vi "CATPLAT GUI.vi"() -> ()   [LabVIEW 2015]
uses:
  controls/PS3 Controls.ctl
  controls/UDP Message Data.ctl
  <vilib>/Utility/error.llb/DialogType.ctl
  <vilib>/Analysis/baseanly.llb/Mean (DBL).vi
  <vilib>/Instr/_visa.llb/VISA Configure Serial Port (Instr).vi
  <vilib>/Instr/_visa.llb/VISA Configure Serial Port (Serial Instr).vi
  <vilib>/Utility/inputDevices.llb/closeJoystick.vi
  <vilib>/regexp/Match Regular Expression.xnode
  <vilib>/Analysis/NI_AALBase.lvlib
panel:
  out "Change PWM":bool
  out "Serial Ports Number":u32
  out "semSocket":T1
  in  "Send ACK":bool
  out "semQueue":T1
  out "UDP Socket":refnum<k16>
  in  "Tab Control":T2(tab)
  out "PWM Indicator":bool caption="PWM"
  out "Speed & Direction":bool
  out "Differential Drive":bool
  out "Righ Caterpillar Speed PWM":i16 caption="Sent Speed Order"
  in  "Right Caterpillar Direction":enum16{"Stop", "Forwards", "Backwards"}(ring) caption="Direction"
  out "Righ Caterpillar Speed":dbl caption="Rcv Speed (m/s)"
  out "Left Caterpillar Speed PWM":i16 caption="Sent Speed Order"
  in  "Left Caterpillar Direction":enum16{"Stop", "Forwards", "Backwards"}(ring) caption="Direction"
  out "Left Caterpillar Speed":dbl caption="Rcv Speed (m/s)"
  out "Sent Exit Command":bool
  in  "Controller Mode":u16(ring) items=["Differential Drive", "Speed & Direction"]
  in  "Exit CATPLAT":bool
  out "CATPLAT Speed (m/s)":dbl(knob) scale=0.0..0.1
  in  "Communication Link":bool
  out "User controller":bool
  out "WiFi Network":bool
  out "UDP Socket":bool
  out "Serial Communication":bool
  in  "stop":bool
  in  "Request Battery":bool
  out "Message received":bool
  out "Error Out":errorcluster
  in  "restart":bool
  out "Battery level":u8(slide) scale=0.0..100.0
  out "rvcMsgs":refnum<queue>
  in  "No. Pulses":i32=8
  in  "Diameter (mm)":i32=10
  in  "PWM":bool
  in  "Threshold":i32=25000
  in  "Message Type":T3(ring)
  out "Change Controller Mode":bool
  in  "Update":bool
  in  "Password":string="caterpillarPlatform"
  in  "SSID":string="caterpillarWiFi"
  in  "Computer  IP":string
  in  "Computer Port":u16=3000
  in  "Platform IP":string
  in  "Platform Port":u16
  out "Left Joystick X Axis":i32
  out "Left Joystick Y Axis":i32
  out "Right Joystick X Axis":i32
  out "Right Joystick Y Axis":i32
  out "PS3 Controls":T4 {"Left Analogue Stick X" scale=-32768.0..32768.0; "Left Analogue Stick Y" scale=32768.0..-32768.0; "Right Analogue Stick X" scale=-32768.0..32768.0; "Right Analogue Stick Y" scale=32768.0..-32768.0; "X Rotation" scale=-32768.0..32768.0; "Y Rotation" scale=-32768.0..32768.0; "L2 Pressure" scale=0.0..32768.0; "Numeric" format="%d°"}
  in  "All Logs":bool
  in  "Clear Log":bool
  in  "Autoscroll":bool=TRUE
  in  "Log":string
  in  "Clear Log Serial":bool
  in  "Autoscroll Serial":bool=TRUE caption="Autoscroll"
  in  "Baud Rate":u32=115200
  in  "Serial Port List":refnum<visa-resource-name>
  in  "Serial log":string
  out "Controller":refnum<k1>
  # "Controls"
  # "Right Caterpillar"
  # "Left Caterpillar"
  # "Errors"
  # "Information"
  # "Controller Settings"
  # "Encoder Settings"
  # "WiFi Network Settings"
  # "UDP Settings"
  # "CATPLAT GUI Log"
  # "CATPLAT Log"
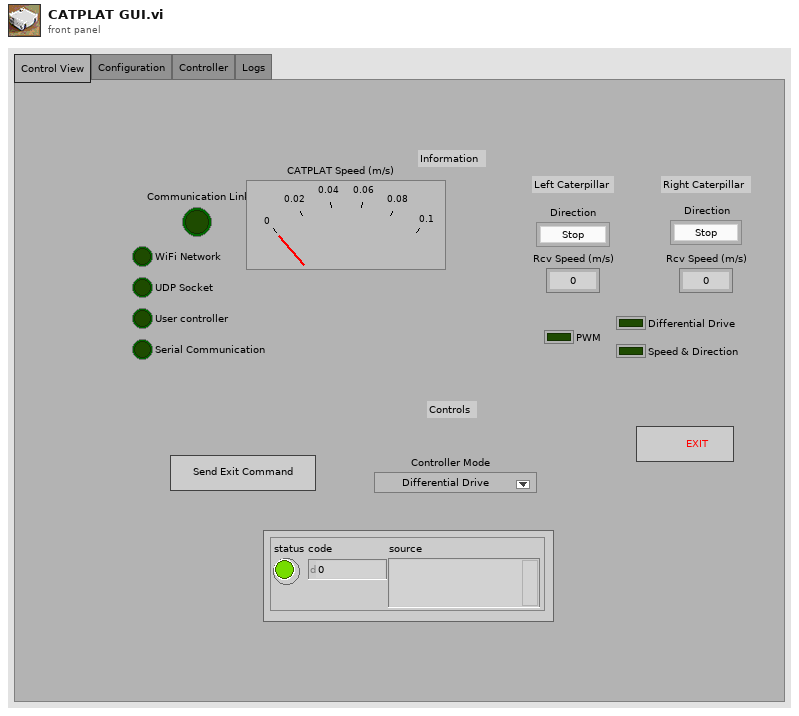
[diagram p1: front panel]
types:
  T1 = typedef "Semaphore RefNum" = refnum<k1>
  T2 = enum32{"Control View", "Configuration", "Controller", "Logs"}
  T3 = enum16{"Acknowledge", "Speed", "Brake", "Watchdog", "Update", "Exit", "Init", "Log", "Unknown"}
  T4 = typedef "PS3 Controls.ctl" = cluster{"Left Analogue Stick X":i32, "Left Analogue Stick Y":i32, "Right Analogue Stick X":i32, "Right Analogue Stick Y":i32, "Y Rotation":i32, "X Rotation":i32, "L2 Pressure":i32, "R2 Pressure":i32, "Triangle":bool, "Circle":bool, "X":bool, "Square":bool, "L1":bool, "R1":bool, "L2":bool, "R2":bool, "L3":bool, "R3":bool, "Select":bool, "Start":bool, "PS Button":bool, "Numeric":i32}
  T5 = enum8{"Enabled", "Disabled", "Disabled and Grayed Out"}
  T6 = typedef "UDP Message Data.ctl" = cluster{"Command":enum16{"Acknowledge", "Speed", "Brake", "Watchdog", "Update", "Exit", "Init", "Log", "Unknown"}, "Msg Length":u8, "Content Bytes":u8[], "Content String":string, "CRC8":u8, "Valid?":bool}
  T7 = typedef "DialogType.ctl" = u16
  T8 = enum32{"invalid app kind", "Development System", "Run Time System", "Student Edition", "Embedded LabVIEW", "Evaluation", "Custom"}
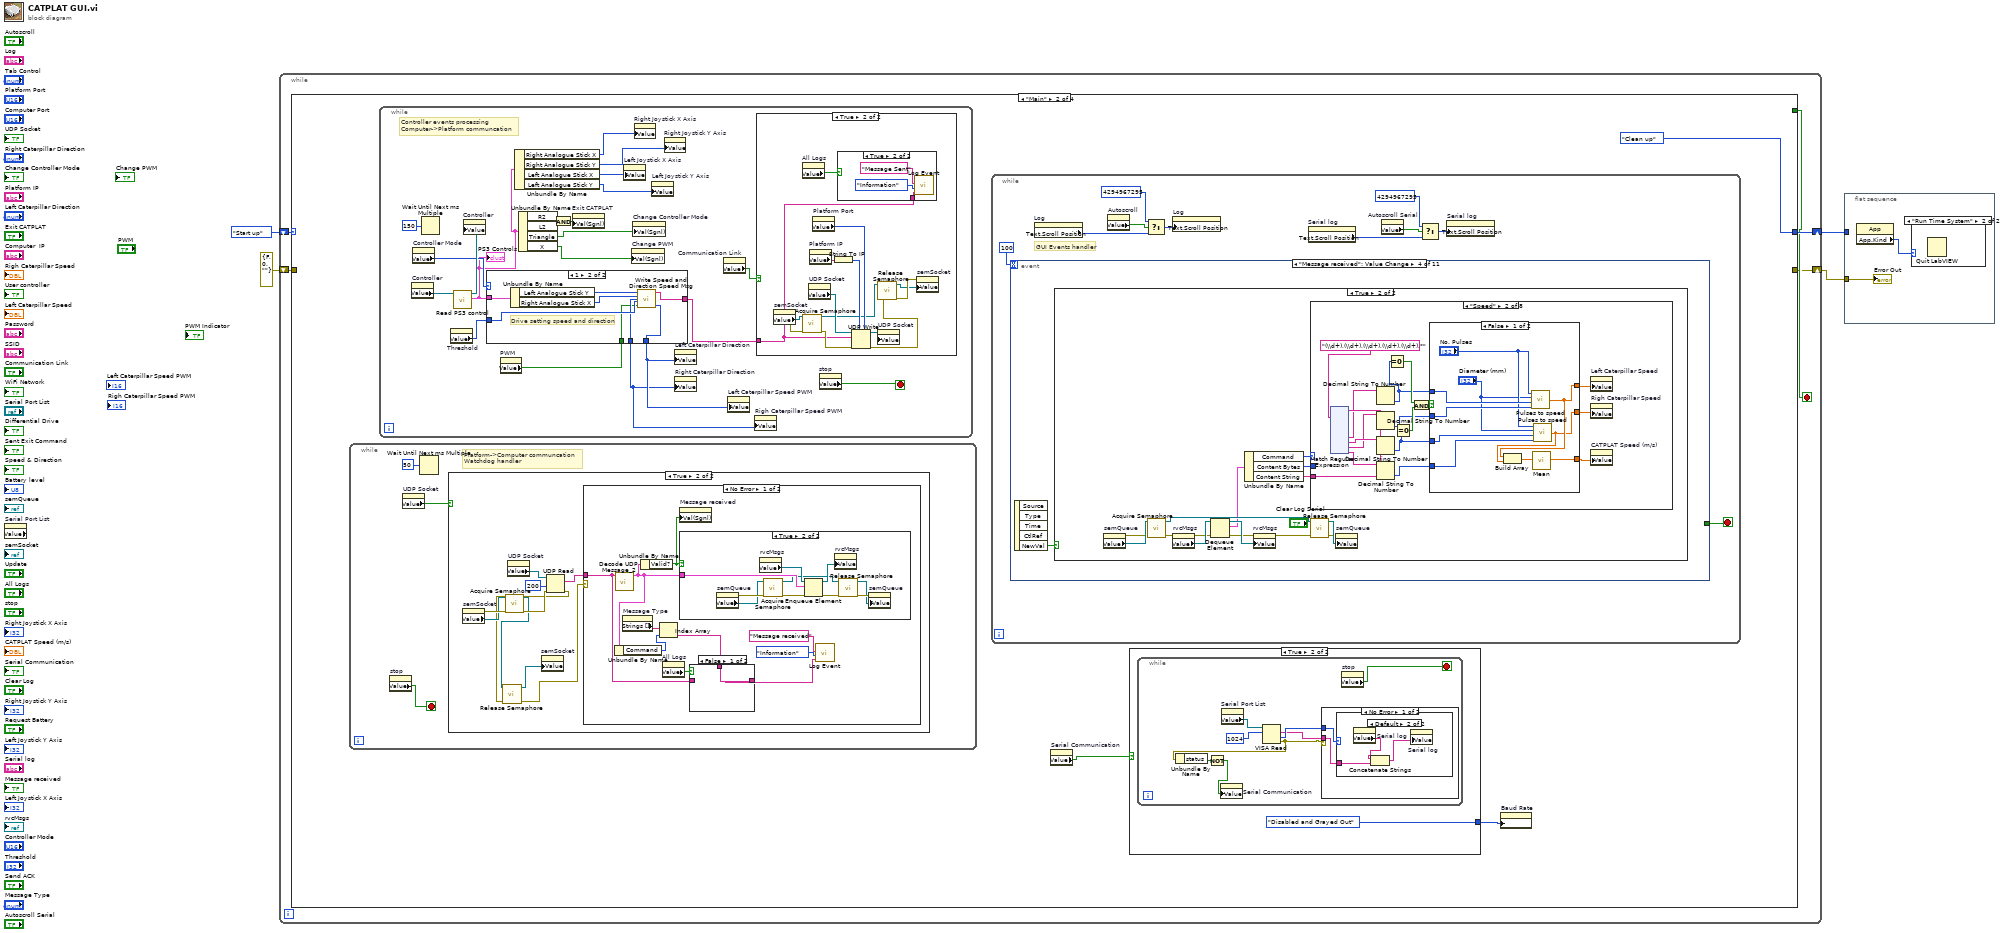
[diagram p0: block diagram]
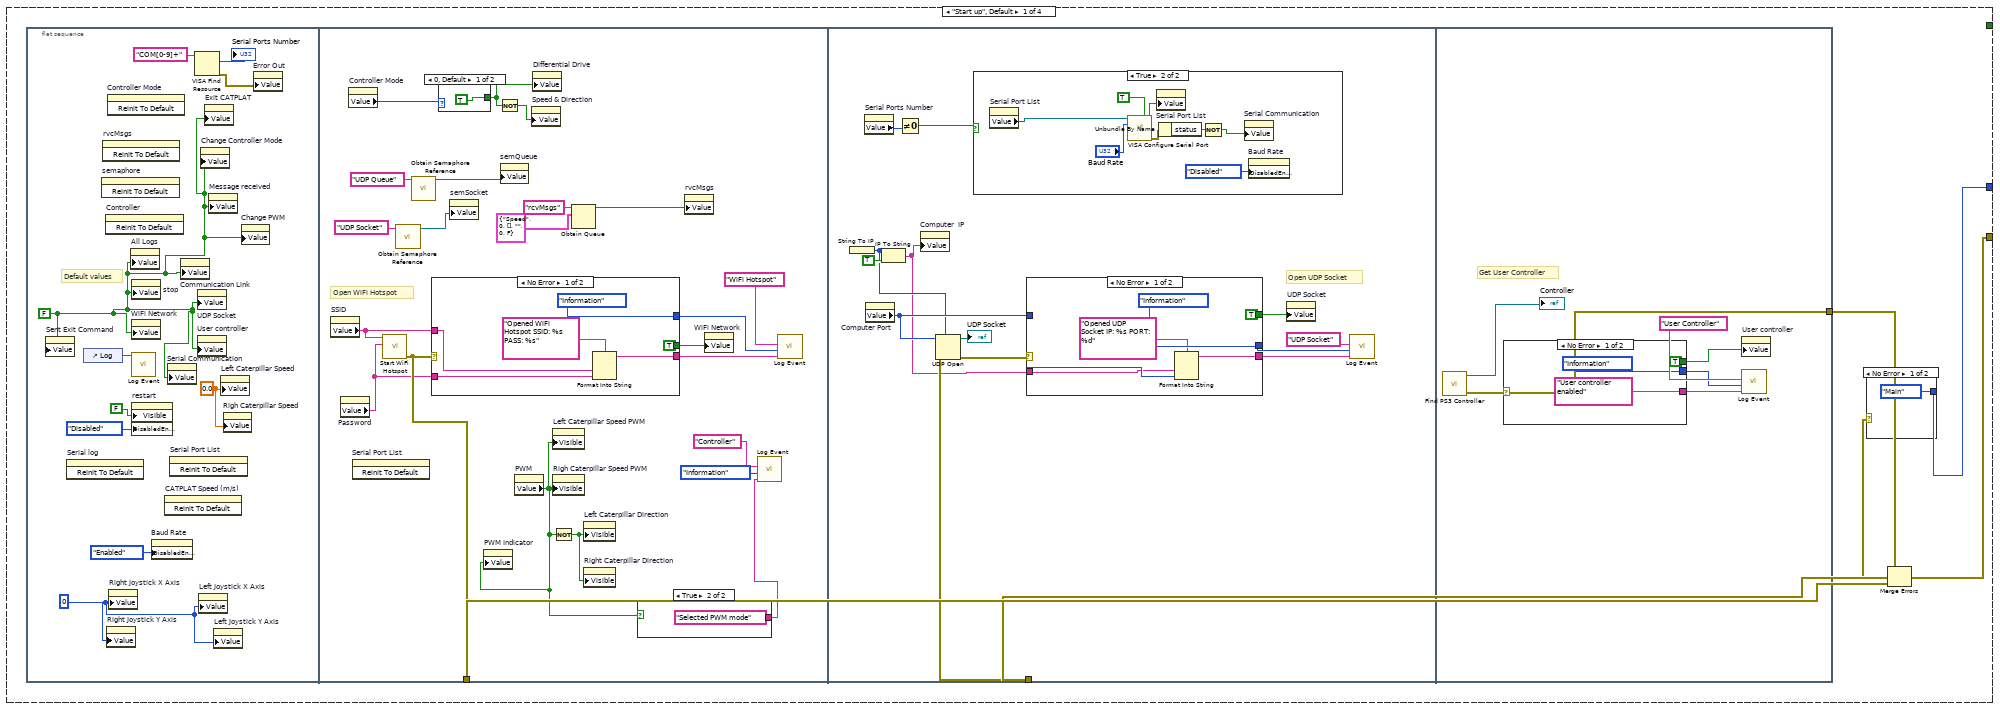
[diagram p3: hidden frame]
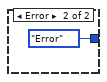
[diagram p4: hidden frame]
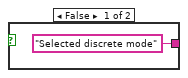
[diagram p5: hidden frame]
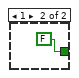
[diagram p6: hidden frame]
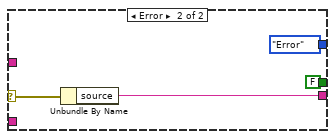
[diagram p7: hidden frame]
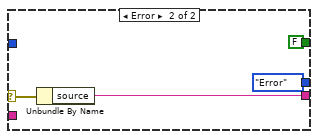
[diagram p9: hidden frame]
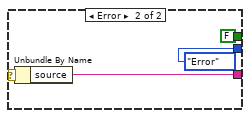
[diagram p10: hidden frame]
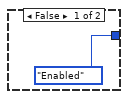
[diagram p11: hidden frame]
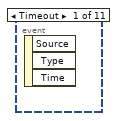
[diagram p14: hidden frame]
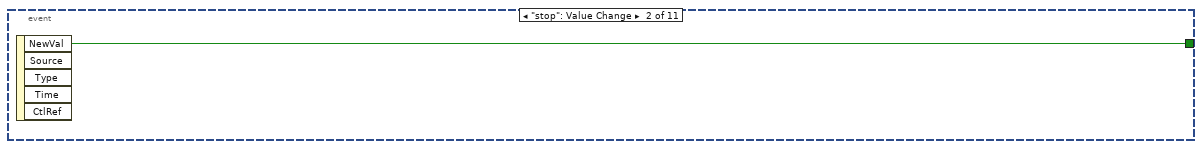
[diagram p15: hidden frame]
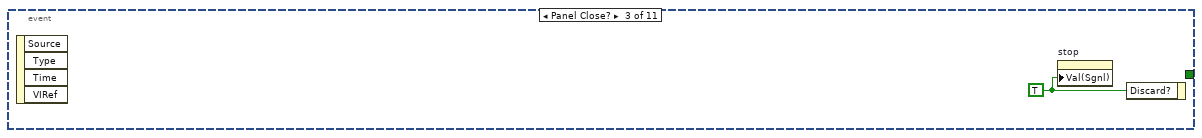
[diagram p16: hidden frame]
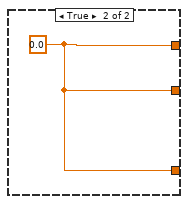
[diagram p19: hidden frame]
diagram:
  n1 = property on="Serial Port List" class="VISAName" props=["Value"]() -> ()  [unwired: 2 in, 3 out]
  n2 = while {
    shift-right: [w8] -> w3
    shift-left: enum16{"Start up", "Error", "Main", "Clean up"}."Start up" -> [w9]
    shift-right: [w6] -> w2
    shift-left: errorcluster {"status"=FALSE, "code"=0, "source"=""} ("error IO") -> [w5]
    stop <- w7 stop-if-true
    n3 = case shown="\"Main\"" w9 {
      selector: w9 -> [_ _ w634 _]
      tunnel: [w14 enum16{"Start up", "Error", "Main", "Clean up"}."Clean up" w634 w641] -> w8
      tunnel: [_ _ TRUE _] -> w7
      tunnel: [w10 _ w628 errorcluster {"status"=FALSE, "code"=0, "source"=""} ("error IO")] -> w6
      tunnel: w5 -> [_ _ w627 w640]
      frame "Start up", Default {
        n4 = flat-sequence {
          tunnel: [w48] -> w12
          tunnel: [w73] -> w11
          tunnel: [w93] -> w13
          frame #0 {
            w18 = i64 0 ("Right Joystick X Axis")
            w23 = 0.0 ("Left wheel speed")
            w17 = FALSE ("stop")
            # "Default values"
            n5 = property on="Sent Exit Command" class="Bool (strict)"("Value"=w17) -> ()  [unwired: 2 in, 2 out]
            n6 = invoke on="Serial log" class="Str" method="Reinit To Default"() -> ()  [unwired: 3 in, 3 out]
            n7 = control-ref of="Log"() -> (w24:refnum<vi>)
            n8 = invoke on="semaphore" class="TypRef (strict)" method="Reinit To Default"() -> ()  [unwired: 3 in, 3 out]
            n9 = invoke on="rvcMsgs" class="TypRef (strict)" method="Reinit To Default"() -> ()  [unwired: 3 in, 3 out]
            n10 = invoke on="Controller" class="TypRef (strict)" method="Reinit To Default"() -> ()  [unwired: 3 in, 3 out]
            n11 = property on="Right Joystick Y Axis" class="DigNum (strict)"("Value"=w18) -> ()  [unwired: 2 in, 2 out]
            n12 = invoke on="Controller Mode" class="Ring (strict)" method="Reinit To Default"() -> ()  [unwired: 3 in, 3 out]
            n13 = property on="Right Joystick X Axis" class="DigNum (strict)"("Value"=w18) -> ()  [unwired: 2 in, 2 out]
            n14 = property on="All Logs" class="Bool (strict)"("Value"=w17) -> ()  [unwired: 2 in, 2 out]
            n15 = property on="stop" class="Bool (strict)"("Value"=w17) -> ()  [unwired: 2 in, 2 out]
            n16 = property on="WiFi Network" class="Bool (strict)"("Value"=w17) -> ()  [unwired: 2 in, 2 out]
            n17 = call "Log Event.vi"("Log Refnum"=w24) -> ()  [unwired: 11 in]
            n18 = property on="restart" class="Bool (strict)"("Visible"=FALSE, "DisabledEnum"=T5."Disabled" ("Disabled")) -> ()  [unwired: 2 in, 2 out]
            n19 = property on="Baud Rate" class="DigNum (strict)"("DisabledEnum"=T5."Enabled" ("Disabled")) -> ()  [unwired: 2 in, 2 out]
            n20 = invoke on="CATPLAT Speed (m/s)" class="Knob (strict)" method="Reinit To Default"() -> ()  [unwired: 3 in, 3 out]
            n21 = property on="Serial Communication" class="Bool (strict)"("Value"=w17) -> ()  [unwired: 2 in, 2 out]
            n22 = invoke on="Serial Port List" class="VISAName" method="Reinit To Default"() -> ()  [unwired: 3 in, 3 out]
            n23 = property on="Communication Link" class="Bool (strict)"("Value"=w17) -> ()  [unwired: 2 in, 2 out]
            n24 = VISA Find Resource(11:"COM[0-9]+" ("expression (\"?*\")")) -> (0:w20:errorcluster, 2:→"Serial Ports Number":u32)  [unwired: 2 in, 1 out]
            n25 = property on="UDP Socket" class="Bool (strict)"("Value"=w17) -> ()  [unwired: 2 in, 2 out]
            n26 = property on="User controller" class="Bool (strict)"("Value"=w17) -> ()  [unwired: 2 in, 2 out]
            n27 = property on="Left Joystick X Axis" class="DigNum (strict)"("Value"=w18) -> ()  [unwired: 2 in, 2 out]
            n28 = property on="Change Controller Mode" class="Bool (strict)"("Value"=w17) -> ()  [unwired: 2 in, 2 out]
            n29 = property on="Exit CATPLAT" class="Bool (strict)"("Value"=w17) -> ()  [unwired: 2 in, 2 out]
            n30 = property on="Message received" class="Bool (strict)"("Value"=w17) -> ()  [unwired: 2 in, 2 out]
            n31 = property on="Left Joystick Y Axis" class="DigNum (strict)"("Value"=w18) -> ()  [unwired: 2 in, 2 out]
            n32 = property on="Left Caterpillar Speed" class="DigNum (strict)"("Value"=w23) -> ()  [unwired: 2 in, 2 out]
            n33 = property on="Righ Caterpillar Speed" class="DigNum (strict)"("Value"=w23) -> ()  [unwired: 2 in, 2 out]
            n34 = property on="Change PWM" class="Bool (strict)"("Value"=w17) -> ()  [unwired: 2 in, 2 out]
            n35 = property on="Error Out" class="Clust (strict)"("Value"=w20) -> ()  [unwired: 2 in, 2 out]
          }
          frame #1 {
            # "Open WiFi Hotspot"
            n36 = property on="SSID" class="Str"() -> ("Value"=w46:string)  [unwired: 2 in, 2 out]
            n37 = property on="Password" class="Str"() -> ("Value"=w45:string)  [unwired: 2 in, 2 out]
            n38 = property on="Controller Mode" class="Ring (strict)"() -> ("Value"=w34:u16)  [unwired: 2 in, 2 out]
            n39 = invoke on="Serial Port List" class="VISAName" method="Reinit To Default"() -> ()  [unwired: 3 in, 3 out]
            n40 = call "Start WiFi Hotspot.vi"("Password"=w45, "SSID"=w46) -> ("error out"=w48:errorcluster)  [unwired: 9 in]
            n41 = call <vilib>:"Obtain Semaphore Reference.vi"("name (unnamed)"="UDP Socket") -> ("semaphore"=w35:T1)  [unwired: 4 in, 2 out]
            n42 = call <vilib>:"Obtain Semaphore Reference.vi"("name (unnamed)"="UDP Queue") -> ("semaphore"=w36:T1)  [unwired: 4 in, 2 out]
            n43 = case shown="No Error" w48 {
              selector: w48 -> [_ w61]
              tunnel: [enum16{"Information", "Warning", "Error"}."Information" ("Enum") enum16{"Information", "Warning", "Error"}."Error" ("Enum")] -> w47
              tunnel: w46 -> [w56 _]
              tunnel: w45 -> [w55 _]
              tunnel: [w54 w60] -> w44
              tunnel: [TRUE ("WiFi Network") FALSE ("WiFi Network")] -> w42
              frame No Error {
                n44 = Format Into String(format string="Opened WiFi Hotspot SSID: %s PASS: %s" ("Event"), w56, w55) -> (resulting string=w54:string)  [unwired: 2 in, 1 out]
              }
              frame Error {
                n45 = Unbundle By Name(w61) -> ("source"=w60:string)
              }
            }
            n46 = case shown="0, Default" w34 {
              tunnel: [TRUE FALSE] -> w33
              frame 0, Default {
              }
              frame 1 {
              }
            }
            n47 = property on="semSocket" class="TypRef (strict)"("Value"=w35) -> ()  [unwired: 2 in, 2 out]
            n48 = Not(x=w33) -> (.not. x?=w32:bool)
            n49 = property on="semQueue" class="TypRef (strict)"("Value"=w36) -> ()  [unwired: 2 in, 2 out]
            n50 = property on="PWM" class="Bool (strict)"() -> ("Value"=w27:bool)  [unwired: 2 in, 2 out]
            n51 = property on="PWM Indicator" class="Bool (strict)"("Value"=w27) -> ()  [unwired: 2 in, 2 out]
            n52 = property on="Speed & Direction" class="Bool (strict)"("Value"=w32) -> ()  [unwired: 2 in, 2 out]
            n53 = property on="Differential Drive" class="Bool (strict)"("Value"=w33) -> ()  [unwired: 2 in, 2 out]
            n54 = Not(x=w27) -> (.not. x?=w31:bool)
            n55 = property on="Left Caterpillar Speed PWM" class="DigNum (strict)"("Visible"=w27) -> ()  [unwired: 2 in, 2 out]
            n56 = property on="Righ Caterpillar Speed PWM" class="DigNum (strict)"("Visible"=w27) -> ()  [unwired: 2 in, 2 out]
            n57 = Obtain Queue(name (unnamed)="rcvMsgs", element data type=T6 {"Command"=enum."Speed", "Msg Length"=0, "Content Bytes"=[], "Content String"="", "CRC8"=0, "Valid?"=FALSE} ("Data")) -> (queue out=w40:refnum<queue>)  [unwired: 3 in, 2 out]
            n58 = property on="Left Caterpillar Direction" class="Enum (strict)"("Visible"=w31) -> ()  [unwired: 2 in, 2 out]
            n59 = property on="Right Caterpillar Direction" class="Enum (strict)"("Visible"=w31) -> ()  [unwired: 2 in, 2 out]
            n60 = case shown="True" w27 {
              tunnel: ["Selected discrete mode" ("Event") "Selected PWM mode" ("Event")] -> w28
              frame False {
              }
              frame True {
              }
            }
            n61 = property on="rvcMsgs" class="TypRef (strict)"("Value"=w40) -> ()  [unwired: 2 in, 2 out]
            n62 = property on="WiFi Network" class="Bool (strict)"("Value"=w42) -> ()  [unwired: 2 in, 2 out]
            n63 = call "Log Event.vi"("Event"=w28, "Enum"=enum16{"Information", "Warning", "Error"}."Information", "Process"="Controller") -> ()  [unwired: 9 in]
            n64 = call "Log Event.vi"("Event"=w44, "Enum"=w47, "Process"="WiFi Hotspot") -> ()  [unwired: 9 in]
          }
          frame #2 {
            # "Open UDP Socket"
            n65 = String To IP() -> (0:w66:u32)  [unwired: 1 in]
            n66 = property on="Serial Ports Number" class="DigNum (strict)"() -> ("Value"=w64:u32)  [unwired: 2 in, 2 out]
            n67 = property on="Computer Port" class="DigNum (strict)"() -> ("Value"=w72:u16)  [unwired: 2 in, 2 out]
            n68 = IP To String(1:TRUE ("dot notation? (F)"), 2:w66) -> (0:w65:string)
            n69 = Not Equal To 0?(x=w64) -> (x != 0?=w63:bool)
            n70 = property on="Computer  IP" class="Str"("Value"=w65) -> ()  [unwired: 2 in, 2 out]
            n71 = UDP Open(7:w66, 11:w72) -> (port=→"UDP Socket":refnum<k16>, 0:w73:errorcluster)  [unwired: 3 in, 1 out]
            n72 = case shown="True" w63 {
              frame False {
              }
              frame True {
                n73 = property on="Serial Port List" class="VISAName"() -> ("Value"=w79:refnum<visa-resource-name>)  [unwired: 2 in, 2 out]
                n74 = call-poly "VISA Configure Serial Port"("VISA resource name"=w79, "Enable Termination\nChar (T)"=TRUE ("Enable Termination\nChar (T)"), "baud rate (9600)"="Baud Rate") -> ("VISA resource name out"=w80:refnum<visa-resource-name>, "error out"=w77:errorcluster)  [unwired: 11 in]
                n75 = property on="Serial Port List" class="VISAName"("Value"=w80) -> ()  [unwired: 2 in, 2 out]
                n76 = Unbundle By Name(w77) -> ("status"=w76:bool)
                n77 = Not(x=w76) -> (.not. x?=w75:bool)
                n78 = property on="Serial Communication" class="Bool (strict)"("Value"=w75) -> ()  [unwired: 2 in, 2 out]
                n79 = property on="Baud Rate" class="DigNum (strict)"("DisabledEnum"=T5."Disabled" ("Disabled")) -> ()  [unwired: 2 in, 2 out]
              }
            }
            n80 = case shown="No Error" w73 {
              selector: w73 -> [_ w91]
              tunnel: [enum16{"Information", "Warning", "Error"}."Information" ("Enum") enum16{"Information", "Warning", "Error"}."Error" ("Enum")] -> w70
              tunnel: w72 -> [w85 _]
              tunnel: w65 -> [w84 _]
              tunnel: [w86 w90] -> w71
              tunnel: [TRUE ("UDP Communication") FALSE ("UDP Communication")] -> w68
              frame No Error {
                n81 = Format Into String(format string="Opened UDP Socket IP: %s PORT: %d" ("Event"), w84, w85) -> (resulting string=w86:string)  [unwired: 2 in, 1 out]
              }
              frame Error {
                n82 = Unbundle By Name(w91) -> ("source"=w90:string)
              }
            }
            n83 = property on="UDP Socket" class="Bool (strict)"("Value"=w68) -> ()  [unwired: 2 in, 2 out]
            n84 = call "Log Event.vi"("Event"=w71, "Enum"=w70, "Process"="UDP Socket") -> ()  [unwired: 9 in]
          }
          frame #3 {
            # "Get User Controller"
            n85 = call "Find PS3 Controller.vi"() -> ("error out"=w93:errorcluster, "Controller Reference Out"=→"Controller":refnum<k1>)  [unwired: 10 in]
            n86 = case shown="No Error" w93 {
              selector: w93 -> [_ w104]
              tunnel: [enum16{"Information", "Warning", "Error"}."Information" ("Enum") enum16{"Information", "Warning", "Error"}."Error" ("Enum")] -> w95
              tunnel: ["User controller enabled" ("Event") w103] -> w97
              tunnel: [TRUE ("UDP Communication") FALSE ("UDP Communication")] -> w98
              frame No Error {
              }
              frame Error {
                n87 = Unbundle By Name(w104) -> ("source"=w103:string)
              }
            }
            n88 = property on="User controller" class="Bool (strict)"("Value"=w98) -> ()  [unwired: 2 in, 2 out]
            n89 = call "Log Event.vi"("Event"=w97, "Enum"=w95, "Process"="User Controller") -> ()  [unwired: 9 in]
          }
        }
        n90 = Merge Errors(w13, w11, w12) -> (w10:errorcluster)
        n91 = case shown="No Error" w10 {
          tunnel: [enum16{"Start up", "Error", "Main", "Clean up"}."Main" enum16{"Start up", "Error", "Main", "Clean up"}."Error"] -> w14
          frame No Error {
          }
          frame Error {
          }
        }
      }
      frame "Main" {
        n92 = while {
          stop <- w583 stop-if-true
          # "Platform->Computer communcation\nWatchdog handler"
          n93 = property on="stop" class="Bool (strict)"() -> ("Value"=w583:bool)  [unwired: 2 in, 2 out]
          n94 = property on="UDP Socket" class="Bool (strict)"() -> ("Value"=w585:bool)  [unwired: 2 in, 2 out]
          n95 = Wait Until Next ms Multiple(millisecond multiple=u32 50) -> ()  [unwired: 1 out]
          n96 = case shown="True" w585 {
            frame False {
            }
            frame True {
              n97 = property on="semSocket" class="TypRef (strict)"() -> (error out=w592:errorcluster, "Value"=w591:T1)  [unwired: 2 in, 1 out]
              n98 = call <vilib>:"Acquire Semaphore.vi"("error in (no error)"=w592, "semaphore"=w591) -> ("error out"=w590:errorcluster, "semaphore out"=w588:T1)  [unwired: 3 in, 1 out]
              n99 = property on="UDP Socket" class="Ref (strict)"() -> ("Value"=w595:refnum<k16>)  [unwired: 2 in, 2 out]
              n100 = UDP Read(connection ID=w595, timeout ms (25000)=200, 8:w590) -> (data out=w593:string, error out=w587:errorcluster)  [unwired: 1 in, 3 out]
              n101 = call <vilib>:"Release Semaphore.vi"("error in (no error)"=w587, "semaphore"=w588) -> ("error out"=w586:errorcluster, "semaphore out"=w589:T1)  [unwired: 4 in]
              n102 = property on="semSocket" class="TypRef (strict)"("Value"=w589) -> ()  [unwired: 2 in, 2 out]
              n103 = case shown="No Error" w586 {
                tunnel: w593 -> [w601 _]
                frame No Error {
                  n104 = call "Decode UDP Message_2.vi"("Input string"=w601) -> ("Data"=w597:T6)  [unwired: 10 in]
                  n105 = Unbundle By Name(w597) -> ("Command"=w598:T3)
                  n106 = property on="Message Type" class="Enum (strict)"() -> ("Strings []"=w599:string[])  [unwired: 2 in, 2 out]
                  n107 = Unbundle By Name(w597) -> ("Valid?"=w603:bool)
                  n108 = Index Array(array=w599, index=w598) -> (element=w596:string)
                  n109 = property on="All Logs" class="Bool (strict)"() -> ("Value"=w602:bool)  [unwired: 2 in, 2 out]
                  n110 = property on="Message received" class="Bool (strict)"("Val(Sgnl)"=w603) -> ()  [unwired: 2 in, 2 out]
                  n111 = case shown="True" w603 {
                    tunnel: w597 -> [_ w617]
                    frame False {
                    }
                    frame True {
                      n112 = property on="semQueue" class="TypRef (strict)"() -> (error out=w616:errorcluster, "Value"=w613:T1)  [unwired: 2 in, 1 out]
                      n113 = property on="rvcMsgs" class="TypRef (strict)"() -> ("Value"=w619:refnum<queue>)  [unwired: 2 in, 2 out]
                      n114 = call <vilib>:"Acquire Semaphore.vi"("error in (no error)"=w616, "semaphore"=w613) -> ("error out"=w611:errorcluster, "semaphore out"=w612:T1)  [unwired: 3 in, 1 out]
                      n115 = Enqueue Element(queue=w619, element=w617, error in (no error)=w611) -> (queue out=w618:refnum<queue>, error out=w610:errorcluster)  [unwired: 1 in, 1 out]
                      n116 = property on="rvcMsgs" class="TypRef (strict)"("Value"=w618) -> ()  [unwired: 2 in, 2 out]
                      n117 = call <vilib>:"Release Semaphore.vi"("error in (no error)"=w610, "semaphore"=w612) -> ("error out"=w615:errorcluster, "semaphore out"=w614:T1)  [unwired: 4 in]
                      n118 = property on="semQueue" class="TypRef (strict)"(error in=w615, "Value"=w614) -> ()  [unwired: 1 in, 2 out]
                    }
                  }
                  n119 = case shown="False" w602 {
                    tunnel: w601 -> [_ w609]
                    tunnel: [w606 w609] -> w600
                    tunnel: w596 -> [w606 w607]
                    frame False {
                    }
                    frame True {
                      n120 = Concatenate Strings(w607, ": " ("string"), w609) -> ()  [unwired: 1 out]
                    }
                  }
                  n121 = call "Log Event.vi"("Event"=w600, "Enum"=enum16{"Information", "Warning", "Error"}."Information", "Process"="Message received") -> ()  [unwired: 9 in]
                }
                frame Error {
                }
              }
            }
          }
        }
        n122 = while {
          stop <- w529 stop-if-true
          # "Controller events processing\nComputer->Platform communcation"
          n123 = property on="Controller" class="TypRef (strict)"() -> ("Value"=w549:refnum<k1>)  [unwired: 2 in, 2 out]
          n124 = property on="Controller Mode" class="Ring (strict)"() -> ("Value"=w547:u16)  [unwired: 2 in, 2 out]
          n125 = Wait Until Next ms Multiple(millisecond multiple=u32 150) -> ()  [unwired: 1 out]
          n126 = property on="Threshold" class="DigNum (strict)"() -> ("Value"=w546:i32)  [unwired: 2 in, 2 out]
          n127 = call "Read PS3 control.vi"("Controller Reference In"=w549) -> ("PS3 Controls"=w538:T4, "Controller Reference Out"=w548:refnum<k1>)  [unwired: 8 in, 1 out]
          "PS3 Controls" <- w538
          n128 = property on="Controller" class="TypRef (strict)"("Value"=w548) -> ()  [unwired: 2 in, 2 out]
          n129 = property on="PWM" class="Bool (strict)"() -> ("Value"=w533:bool)  [unwired: 2 in, 2 out]
          n130 = case shown="1" w547 {
            tunnel: w538 -> [w574 w582]
            tunnel: w546 -> [w573 w581]
            tunnel: [w572 w580] -> w544
            tunnel: [w569 w576] -> w531
            tunnel: [w568 w577] -> w530
            tunnel: w533 -> [w567 w575]
            frame 0, Default {
              # "Drive controlling the caterpillars"
              n131 = Unbundle By Name(w574) -> ("Left Analogue Stick Y"=w571:i32, "Right Analogue Stick Y"=w570:i32)
              n132 = call "Write Differential Speed Msg.vi"("Use PWM?"=w567, "Offset"=w573, "Right Controller Y Axis"=w570, "Left Controller Y Axis"=w571) -> ("Left Motor"=w569:i16, "Right Motor"=w568:i16, "Speed UDP Message"=w572:string)
            }
            frame 1 {
              # "Drive setting speed and direction"
              n133 = Unbundle By Name(w582) -> ("Left Analogue Stick Y"=w579:i32, "Right Analogue Stick X"=w578:i32)
              n134 = call "Write Speed and Direction Speed Msg.vi"("Use PWM?"=w575, "Offset"=w581, "Right Controller X Axis"=w578, "Left Controller Y Axis"=w579) -> ("Left Motor"=w576:i16, "Right Motor"=w577:i16, "Speed UDP Message"=w580:string)
            }
          }
          n135 = Unbundle By Name(w538) -> ("Right Analogue Stick X"=w537:i32, "Right Analogue Stick Y"=w536:i32, "Left Analogue Stick X"=w535:i32, "Left Analogue Stick Y"=w534:i32)
          n136 = Unbundle By Name(w538) -> ("R2"=w541:bool, "L2"=w542:bool, "Triangle"=w539:bool, "X"=w532:bool)
          n137 = And(x=w541, y=w542) -> (x .and. y?=w540:bool)
          n138 = property on="Exit CATPLAT" class="Bool (strict)"("Val(Sgnl)"=w540) -> ()  [unwired: 2 in, 2 out]
          n139 = property on="Left Joystick X Axis" class="DigNum (strict)"("Value"=w535) -> ()  [unwired: 2 in, 2 out]
          n140 = property on="Change PWM" class="Bool (strict)"("Val(Sgnl)"=w532) -> ()  [unwired: 2 in, 2 out]
          n141 = property on="Change Controller Mode" class="Bool (strict)"("Val(Sgnl)"=w539) -> ()  [unwired: 2 in, 2 out]
          n142 = property on="Right Joystick X Axis" class="DigNum (strict)"("Value"=w537) -> ()  [unwired: 2 in, 2 out]
          n143 = property on="Left Joystick Y Axis" class="DigNum (strict)"("Value"=w534) -> ()  [unwired: 2 in, 2 out]
          n144 = property on="Right Joystick Y Axis" class="DigNum (strict)"("Value"=w536) -> ()  [unwired: 2 in, 2 out]
          n145 = property on="Left Caterpillar Direction" class="Enum (strict)"("Value"=w531) -> ()  [unwired: 2 in, 2 out]
          n146 = property on="Right Caterpillar Direction" class="Enum (strict)"("Value"=w530) -> ()  [unwired: 2 in, 2 out]
          n147 = property on="Communication Link" class="Bool (strict)"() -> ("Value"=w543:bool)  [unwired: 2 in, 2 out]
          n148 = property on="Left Caterpillar Speed PWM" class="DigNum (strict)"("Value"=w531) -> ()  [unwired: 2 in, 2 out]
          n149 = property on="Righ Caterpillar Speed PWM" class="DigNum (strict)"("Value"=w530) -> ()  [unwired: 2 in, 2 out]
          n150 = case shown="True" w543 {
            tunnel: w544 -> [_ w550]
            frame False {
            }
            frame True {
              n151 = property on="semSocket" class="TypRef (strict)"() -> (error out=w558:errorcluster, "Value"=w557:T1)  [unwired: 2 in, 1 out]
              n152 = property on="All Logs" class="Bool (strict)"() -> ("Value"=w551:bool)  [unwired: 2 in, 2 out]
              n153 = call <vilib>:"Acquire Semaphore.vi"("error in (no error)"=w558, "semaphore"=w557) -> ("error out"=w553:errorcluster, "semaphore out"=w554:T1)  [unwired: 3 in, 1 out]
              n154 = property on="UDP Socket" class="Ref (strict)"() -> ("Value"=w559:refnum<k16>)  [unwired: 2 in, 2 out]
              n155 = property on="Platform IP" class="Str"() -> ("Value"=w561:string)  [unwired: 2 in, 2 out]
              n156 = property on="Platform Port" class="DigNum (strict)"() -> ("Value"=w563:u16)  [unwired: 2 in, 2 out]
              n157 = String To IP(1:w561) -> (0:w562:u32)
              n158 = case shown="True" w551 {
                tunnel: w550 -> [_ w564]
                frame False {
                }
                frame True {
                  n159 = call "Log Event.vi"("Event"=w564, "Enum"=enum16{"Information", "Warning", "Error"}."Information", "Process"="Message Sent") -> ()  [unwired: 9 in]
                }
              }
              n160 = UDP Write(address=w562, port or service name=w563, connection ID=w559, data in=w550, 8:w553) -> (error out=w552:errorcluster, 3:w560:refnum<k16>)  [unwired: 1 in]
              n161 = call <vilib>:"Release Semaphore.vi"("error in (no error)"=w552, "semaphore"=w554) -> ("error out"=w556:errorcluster, "semaphore out"=w555:T1)  [unwired: 4 in]
              n162 = property on="UDP Socket" class="Ref (strict)"("Value"=w560) -> ()  [unwired: 2 in, 2 out]
              n163 = property on="semSocket" class="TypRef (strict)"(error in=w556, "Value"=w555) -> ()  [unwired: 1 in, 2 out]
            }
          }
          n164 = property on="stop" class="Bool (strict)"() -> ("Value"=w529:bool)  [unwired: 2 in, 2 out]
        }
        n165 = while {
          stop <- w124 stop-if-true
          # "GUI Events handler"
          n166 = event shown="[3] \"Message received\": Value Change" {
            selector: _ -> [_ _ _ _ _ _ _ _ _ _ _]
            dyn-events: _ -> [_ _ _ _ _ _ _ _ _ _ _]
            timeout: 100 -> [_ _ _ _ _ _ _ _ _ _ _]
            tunnel: [_ w134 _ _ _ _ _ _ _ _ _] -> w124
            event Timeout {
              n167 = event-data() -> ()  [unwired: 1 in, 3 out]
            }
            event "stop": Value Change {
              n168 = event-data() -> ("NewVal"=w134:bool)  [unwired: 1 in, 4 out]
            }
            event Panel Close? {
              w135 = TRUE ("Discard?")
              n169 = event-data() -> ()  [unwired: 1 in, 4 out]
              n170 = property on="stop" class="Bool (strict)"("Val(Sgnl)"=w135) -> ()  [unwired: 2 in, 2 out]
              n171 = event-data("Discard?"=w135) -> ()  [unwired: 1 in, 1 out]
            }
            event "Message received": Value Change {
              n172 = event-data() -> ("NewVal"=w136:bool)  [unwired: 1 in, 4 out]
              n173 = case shown="True" w136 {
                frame False {
                }
                frame True {
                  n174 = property on="semQueue" class="TypRef (strict)"() -> (error out=w144:errorcluster, "Value"=w148:T1)  [unwired: 2 in, 1 out]
                  n175 = call <vilib>:"Acquire Semaphore.vi"("error in (no error)"=w144, "semaphore"=w148) -> ("error out"=w149:errorcluster, "semaphore out"=w141:T1)  [unwired: 3 in, 1 out]
                  n176 = property on="rvcMsgs" class="TypRef (strict)"(error in=w149) -> (error out=w143:errorcluster, "Value"=w150:refnum<queue>)  [unwired: 1 in, 1 out]
                  n177 = Dequeue Element(queue=w150, error in (no error)=w143) -> (queue out=w151:refnum<queue>, element=w140:T6, error out=w142:errorcluster)  [unwired: 1 in, 1 out]
                  n178 = Unbundle By Name(w140) -> ("Command"=w139:T3, "Content Bytes"=w138:u8[], "Content String"=w137:string)
                  n179 = property on="rvcMsgs" class="TypRef (strict)"(error in=w142, "Value"=w151) -> (error out=w147:errorcluster)  [unwired: 1 in, 1 out]
                  n180 = case shown="\"Speed\"" w139 {
                    tunnel: w138 -> [_ _ _ _ _ _ _ _]
                    tunnel: w137 -> [_ w167 _ _ _ w304 _ _]
                    frame "Acknowledge", Default {
                    }
                    frame "Speed" {
                      n181 = xnode "Match Regular Expression"("input string"=w167, "regular expression"="(\\d+),(\\d+),(\\d+),(\\d+),(\\d+).*") -> ("submatch 2"=w165:string, "submatch 3"=w164:string, "submatch 4"=w163:string, "submatch 5"=w162:string)  [unwired: 4 in, 6 out]
                      n182 = Decimal String To Number(string=w165) -> (number=w152:i32)  [unwired: 2 in, 1 out]
                      n183 = Decimal String To Number(string=w163) -> (number=w153:i32)  [unwired: 2 in, 1 out]
                      n184 = Decimal String To Number(string=w164) -> (number=w154:i32)  [unwired: 2 in, 1 out]
                      n185 = Decimal String To Number(string=w162) -> (number=w155:i32)  [unwired: 2 in, 1 out]
                      n186 = Equal To 0?(x=w152) -> (x = 0?=w157:bool)
                      n187 = Equal To 0?(x=w154) -> (x = 0?=w156:bool)
                      n188 = And(x=w157, y=w156) -> (x .and. y?=w158:bool)
                      n189 = case shown="False" w158 {
                        tunnel: w152 -> [w176 _]
                        tunnel: w153 -> [w175 _]
                        tunnel: w154 -> [w174 _]
                        tunnel: w155 -> [w173 _]
                        tunnel: [w177 w178] -> w161
                        tunnel: [w170 w178] -> w160
                        tunnel: [w169 w178] -> w159
                        frame False {
                          n190 = call "Pulses to speed.vi"("Elapsed time (ms)"=w175, "Pulses"=w176, "Enc. Diameter (mm)"="Diameter (mm)", "No. pulses/rev"="No. Pulses") -> ("Speed (m/s)"=w170:dbl)
                          n191 = call "Pulses to speed.vi"("Elapsed time (ms)"=w173, "Pulses"=w174, "Enc. Diameter (mm)"="Diameter (mm)", "No. pulses/rev"="No. Pulses") -> ("Speed (m/s)"=w169:dbl)
                          n192 = Build Array(w170, w169) -> (w168:dbl[])
                          n193 = call-poly <vilib>:"Mean.vi"("X"=w168) -> ("mean"=w177:dbl)  [unwired: 1 out]
                        }
                        frame True {
                          w178 = 0.0
                        }
                      }
                      n194 = property on="Left Caterpillar Speed" class="DigNum (strict)"("Value"=w160) -> ()  [unwired: 2 in, 2 out]
                      n195 = property on="Righ Caterpillar Speed" class="DigNum (strict)"("Value"=w159) -> ()  [unwired: 2 in, 2 out]
                      n196 = property on="CATPLAT Speed (m/s)" class="Knob (strict)"("Value"=w161) -> ()  [unwired: 2 in, 2 out]
                    }
                    frame "Brake" {
                    }
                    frame "Watchdog" {
                    }
                    frame "Update" {
                    }
                    frame "Init" {
                      n197 = xnode "Match Regular Expression"("input string"=w304, "regular expression"="(\\d+)@(\\d{1,3}.\\d{1,3}.\\d{1,3}.\\d{1,3})") -> ("submatch 1"=w303:string, "submatch 2"=w301:string)  [unwired: 4 in, 5 out]
                      n198 = String To IP(1:w301) -> (0:w315:u32)
                      n199 = IP To String(1:TRUE ("dot notation? (F)"), 2:w315) -> (0:w313:string)
                      n200 = Decimal String To Number(string=w303, default (0L)=i16 0 ("default (0 I32)")) -> (number=w302:i16)  [unwired: 1 in, 1 out]
                      n201 = Equal?(x=w313, y=w301) -> (x = y?=w299:bool)
                      n202 = case shown="False" w299 {
                        tunnel: [enum16{"Information", "Warning", "Error"}."Error" ("Enum") enum16{"Information", "Warning", "Error"}."Information" ("Enum")] -> w308
                        tunnel: w304 -> [_ w436]
                        tunnel: ["CATPLAT Invalid IP" w435] -> w307
                        frame False {
                        }
                        frame True {
                          n203 = Concatenate Strings("CATPLAT:" ("Event"), w436) -> (w435:string)
                        }
                      }
                      n204 = Select(t=w302, s=w299, f=i16 0) -> (s? t:f=w309:i16)
                      n205 = Select(t=w301, s=w299, f="") -> (s? t:f=w311:string)
                      n206 = property on="Send ACK" class="Bool (strict)"("Val(Sgnl)"=w299) -> ()  [unwired: 2 in, 2 out]
                      n207 = call "Log Event.vi"("Event"=w307, "Enum"=w308, "Process"="Init Comms") -> ()  [unwired: 9 in]
                      n208 = property on="Platform Port" class="DigNum (strict)"("Value"=w309) -> ()  [unwired: 2 in, 2 out]
                      n209 = property on="Platform IP" class="Str"("Value"=w311) -> ()  [unwired: 2 in, 2 out]
                    }
                    frame "Unknown" {
                    }
                    frame "Exit" {
                      n210 = property on="Sent Exit Command" class="Bool (strict)"() -> ("Value"=w439:bool)  [unwired: 2 in, 2 out]
                      n211 = case shown="True" w439 {
                        selector: w439 -> [_ w442]
                        frame False {
                        }
                        frame True {
                          w440 = FALSE ("Communication")
                          n212 = Not(x=w442) -> (.not. x?=w443:bool)
                          n213 = property on="Exit CATPLAT" class="Bool (strict)"("Value"=w443) -> ()  [unwired: 2 in, 2 out]
                          n214 = property on="Communication Link" class="Bool (strict)"("Value"=w440) -> (error out=w441:errorcluster)  [unwired: 2 in, 1 out]
                          n215 = property on="Sent Exit Command" class="Bool (strict)"(error in=w441, "Value"=w440) -> ()  [unwired: 1 in, 2 out]
                          n216 = property on="Send ACK" class="Bool (strict)"("Value"=w440) -> ()  [unwired: 2 in, 2 out]
                          n217 = call "Log Event.vi"("Enum"=enum16{"Information", "Warning", "Error"}."Information", "Process"="ACK exit cmd. End of communications") -> ()  [unwired: 10 in]
                        }
                      }
                    }
                  }
                  n218 = call <vilib>:"Release Semaphore.vi"("error in (no error)"=w147, "semaphore"=w141) -> ("error out"=w145:errorcluster, "semaphore out"=w146:T1)  [unwired: 4 in]
                  n219 = property on="semQueue" class="TypRef (strict)"(error in=w145, "Value"=w146) -> ()  [unwired: 1 in, 2 out]
                }
              }
            }
            event "Change PWM", "PWM": Value Change {
              n220 = event-data() -> ("CtlRef"=w449:refnum<vi>, "OldVal"=w448:bool, "NewVal"=w447:bool)  [unwired: 1 in, 3 out]
              n221 = Exclusive Or(1:w447, 2:w448) -> (0:w446:bool)
              n222 = case shown="True" w446 {
                tunnel: w447 -> [_ w455]
                tunnel: w449 -> [_ w454]
                frame False {
                }
                frame True {
                  n223 = property class="Bool (strict)"(reference=w454) -> ("Label.Text"=w452:string)  [unwired: 1 in, 2 out]
                  n224 = property on="PWM" class="Bool (strict)"() -> ("Label.Text"=w453:string)  [unwired: 2 in, 2 out]
                  n225 = Equal?(x=w452, y=w453) -> (x = y?=w451:bool)
                  n226 = case shown="False" w451 {
                    tunnel: [w461 w465] -> w450
                    tunnel: w455 -> [w460 w465]
                    frame False {
                      n227 = case shown="False" w460 {
                        tunnel: [w462 w463] -> w461
                        frame False {
                          n228 = property on="PWM" class="Bool (strict)"() -> ("Value"=w462:bool)  [unwired: 2 in, 2 out]
                        }
                        frame True {
                          n229 = property on="PWM" class="Bool (strict)"() -> ("Value"=w464:bool)  [unwired: 2 in, 2 out]
                          n230 = Not(x=w464) -> (.not. x?=w463:bool)
                        }
                      }
                    }
                    frame True {
                    }
                  }
                  n231 = property on="PWM" class="Bool (strict)"("Value"=w450) -> ()  [unwired: 2 in, 2 out]
                  n232 = Not(x=w450) -> (.not. x?=w456:bool)
                  n233 = property on="PWM Indicator" class="Bool (strict)"("Value"=w450) -> ()  [unwired: 2 in, 2 out]
                  n234 = case shown="True" w450 {
                    tunnel: ["Selected discrete mode" ("Event") "Selected PWM mode" ("Event")] -> w457
                    frame False {
                    }
                    frame True {
                    }
                  }
                  n235 = property on="Left Caterpillar Direction" class="Enum (strict)"("Visible"=w456) -> ()  [unwired: 2 in, 2 out]
                  n236 = property on="Right Caterpillar Direction" class="Enum (strict)"("Visible"=w456) -> ()  [unwired: 2 in, 2 out]
                  n237 = property on="Left Caterpillar Speed PWM" class="DigNum (strict)"("Visible"=w450) -> ()  [unwired: 2 in, 2 out]
                  n238 = property on="Righ Caterpillar Speed PWM" class="DigNum (strict)"("Visible"=w450) -> ()  [unwired: 2 in, 2 out]
                  n239 = call "Log Event.vi"("Event"=w457, "Enum"=enum16{"Information", "Warning", "Error"}."Information", "Process"="Controller") -> ()  [unwired: 9 in]
                }
              }
            }
            event "Send ACK": Value Change {
              n240 = event-data() -> ("NewVal"=w468:bool)  [unwired: 1 in, 5 out]
              n241 = case shown="False" w468 {
                frame False {
                }
                frame True {
                  n242 = property on="semSocket" class="TypRef (strict)"() -> (error out=w472:errorcluster, "Value"=w480:T1)  [unwired: 2 in, 1 out]
                  n243 = call <vilib>:"Acquire Semaphore.vi"("error in (no error)"=w472, "semaphore"=w480) -> ("error out"=w477:errorcluster, "semaphore out"=w479:T1)  [unwired: 3 in, 1 out]
                  n244 = property on="UDP Socket" class="Ref (strict)"() -> ("Value"=w482:refnum<k16>)  [unwired: 2 in, 2 out]
                  n245 = property on="Platform IP" class="Str"() -> ("Value"=w484:string)  [unwired: 2 in, 2 out]
                  n246 = property on="Platform Port" class="DigNum (strict)"() -> ("Value"=w486:u16)  [unwired: 2 in, 2 out]
                  n247 = String To IP(1:w484) -> (0:w485:u32)
                  n248 = UDP Write(address=w485, port or service name=w486, connection ID=w482, data in="ACK", 8:w477) -> (error out=w476:errorcluster, 3:w483:refnum<k16>)  [unwired: 1 in]
                  n249 = property on="UDP Socket" class="Ref (strict)"("Value"=w483) -> ()  [unwired: 2 in, 2 out]
                  n250 = call <vilib>:"Release Semaphore.vi"("error in (no error)"=w476, "semaphore"=w479) -> ("error out"=w473:errorcluster, "semaphore out"=w478:T1)  [unwired: 4 in]
                  n251 = property on="semSocket" class="TypRef (strict)"(error in=w473, "Value"=w478) -> (error out=w474:errorcluster)  [unwired: 1 in, 1 out]
                  n252 = property on="Communication Link" class="Bool (strict)"(error in=w474, "Value"=TRUE ("Communication")) -> ()  [unwired: 1 in, 2 out]
                  n253 = call "Log Event.vi"("Event"="Sent ACK", "Enum"=enum16{"Information", "Warning", "Error"}."Information", "Process"="Comms") -> ()  [unwired: 9 in]
                }
              }
            }
            event "Change Controller Mode": Value Change {
              n254 = event-data() -> ("NewVal"=w487:bool)  [unwired: 1 in, 5 out]
              n255 = case shown="True" w487 {
                frame False {
                }
                frame True {
                  n256 = property on="Controller Mode" class="Ring (strict)"() -> ("Value"=w491:u16)  [unwired: 2 in, 2 out]
                  n257 = case shown="0, Default" w491 {
                    tunnel: [w496 w498] -> w490
                    tunnel: [FALSE TRUE] -> w489
                    frame 0, Default {
                      w496 = u16 1 items=["Differential Drive", "Speed & Direction"] ("Controller Settings")
                    }
                    frame 1 {
                      w498 = u16 0 items=["Differential Drive", "Speed & Direction"] ("Controller Settings")
                    }
                  }
                  n258 = call "Log Event.vi"("Event"="Changed controller mode", "Enum"=enum16{"Information", "Warning", "Error"}."Information", "Process"="Controller") -> ()  [unwired: 9 in]
                  n259 = Not(x=w489) -> (.not. x?=w488:bool)
                  n260 = property on="Controller Mode" class="Ring (strict)"("Value"=w490) -> ()  [unwired: 2 in, 2 out]
                  n261 = property on="Differential Drive" class="Bool (strict)"("Value"=w489) -> ()  [unwired: 2 in, 2 out]
                  n262 = property on="Speed & Direction" class="Bool (strict)"("Value"=w488) -> ()  [unwired: 2 in, 2 out]
                }
              }
            }
            event "Serial Port List": Value Change {
              n263 = event-data() -> ("OldVal"=w506:refnum<visa-resource-name>, "NewVal"=w505:refnum<visa-resource-name>)  [unwired: 1 in, 4 out]
              n264 = VISA Close(VISA resource name=w506) -> (error out=w503:errorcluster)  [unwired: 1 in]
              n265 = property on="Baud Rate" class="DigNum (strict)"() -> ("Value"=w504:u32)  [unwired: 2 in, 2 out]
              n266 = call-poly "VISA Configure Serial Port"("VISA resource name"=w505, "baud rate (9600)"=w504, "error in (no error)"=w503) -> ("error out"=w499:errorcluster)  [unwired: 11 in, 1 out]
              n267 = Unbundle By Name(w499) -> ("status"=w502:bool)
              n268 = property on="Serial log" class="Str"("Value"="") -> ()  [unwired: 2 in, 2 out]
              n269 = Not(x=w502) -> (.not. x?=w501:bool)
              n270 = property on="Serial Communication" class="Bool (strict)"("Value"=w501) -> ()  [unwired: 2 in, 2 out]
            }
            event "Exit CATPLAT": Value Change {
              n271 = event-data() -> ("NewVal"=w507:bool)  [unwired: 1 in, 5 out]
              n272 = case shown="False" w507 {
                selector: w507 -> [_ w508]
                frame False {
                }
                frame True {
                  n273 = property on="semSocket" class="TypRef (strict)"() -> (error out=w516:errorcluster, "Value"=w515:T1)  [unwired: 2 in, 1 out]
                  n274 = property on="Sent Exit Command" class="Bool (strict)"("Value"=w508) -> ()  [unwired: 2 in, 2 out]
                  n275 = property on="UDP Socket" class="Ref (strict)"() -> ("Value"=w512:refnum<k16>)  [unwired: 2 in, 2 out]
                  n276 = call <vilib>:"Acquire Semaphore.vi"("error in (no error)"=w516, "semaphore"=w515) -> ("error out"=w521:errorcluster, "semaphore out"=w522:T1)  [unwired: 3 in, 1 out]
                  n277 = property on="Platform IP" class="Str"() -> ("Value"=w511:string)  [unwired: 2 in, 2 out]
                  n278 = property on="Platform Port" class="DigNum (strict)"() -> ("Value"=w510:u16)  [unwired: 2 in, 2 out]
                  n279 = String To IP(1:w511) -> (0:w524:u32)
                  n280 = UDP Write(address=w524, port or service name=w510, connection ID=w512, data in="X", 8:w521) -> (error out=w520:errorcluster, 3:w509:refnum<k16>)  [unwired: 1 in]
                  n281 = property on="UDP Socket" class="Ref (strict)"("Value"=w509) -> ()  [unwired: 2 in, 2 out]
                  n282 = call <vilib>:"Release Semaphore.vi"("error in (no error)"=w520, "semaphore"=w522) -> ("error out"=w513:errorcluster, "semaphore out"=w514:T1)  [unwired: 4 in]
                  n283 = property on="semSocket" class="TypRef (strict)"(error in=w513, "Value"=w514) -> ()  [unwired: 1 in, 2 out]
                  n284 = call "Log Event.vi"("Event"="Sent Exit cmd", "Enum"=enum16{"Information", "Warning", "Error"}."Information", "Process"="Comms") -> ()  [unwired: 9 in]
                }
              }
            }
            event "Clear Log": Value Change {
              n285 = event-data() -> ("NewVal"=w525:bool)  [unwired: 1 in, 4 out]
              n286 = case shown="True" w525 {
                frame False {
                }
                frame True {
                  n287 = property on="Log" class="Str"("Value"="" ("Log")) -> ()  [unwired: 2 in, 2 out]
                }
              }
            }
            event "Clear Log Serial": Value Change {
              n288 = event-data() -> ("NewVal"=w527:bool)  [unwired: 1 in, 5 out]
              n289 = case shown="True" w527 {
                frame False {
                }
                frame True {
                  n290 = property on="Serial log" class="Str"("Value"="") -> ()  [unwired: 2 in, 2 out]
                }
              }
            }
          }
          n291 = property on="Log" class="Str"() -> ("Text.Scroll Position"=w131:u32)  [unwired: 2 in, 2 out]
          n292 = property on="Autoscroll" class="Bool (strict)"() -> ("Value"=w133:bool)  [unwired: 2 in, 2 out]
          n293 = Select(t=u32 4294967295 ("Text.Scroll Position"), s=w133, f=w131) -> (s? t:f=w130:u32)
          n294 = property on="Log" class="Str"("Text.Scroll Position"=w130) -> ()  [unwired: 2 in, 2 out]
          n295 = property on="Serial log" class="Str"() -> ("Text.Scroll Position"=w127:u32)  [unwired: 2 in, 2 out]
          n296 = property on="Autoscroll Serial" class="Bool (strict)"() -> ("Value"=w125:bool)  [unwired: 2 in, 2 out]
          n297 = Select(t=u32 4294967295 ("Text.Scroll Position"), s=w125, f=w127) -> (s? t:f=w128:u32)
          n298 = property on="Serial log" class="Str"("Text.Scroll Position"=w128) -> ()  [unwired: 2 in, 2 out]
        }
        n299 = property on="Serial Communication" class="Bool (strict)"() -> ("Value"=w108:bool)  [unwired: 2 in, 2 out]
        n300 = case shown="True" w108 {
          tunnel: [T5."Enabled" ("Disabled") T5."Disabled and Grayed Out" ("Disabled")] -> w107
          frame False {
          }
          frame True {
            n301 = while {
              stop <- w112 stop-if-true
              n302 = property on="Serial Port List" class="VISAName"() -> ("Value"=w113:refnum<visa-resource-name>)  [unwired: 2 in, 2 out]
              n303 = VISA Read(VISA resource name=w113, byte count=u32 1024) -> (read buffer=w117:string, return count=w118:u32, error out=w111:errorcluster)  [unwired: 1 in, 1 out]
              n304 = Unbundle By Name(w111) -> ("status"=w115:bool)
              n305 = Not(x=w115) -> (.not. x?=w116:bool)
              n306 = property on="Serial Communication" class="Bool (strict)"("Value"=w116) -> ()  [unwired: 2 in, 2 out]
              n307 = case shown="No Error" w111 {
                tunnel: w117 -> [w120 _]
                tunnel: w118 -> [w119 _]
                frame No Error {
                  n308 = case shown="Default" w119 {
                    tunnel: w120 -> [_ w122]
                    frame 0 {
                    }
                    frame Default {
                      n309 = property on="Serial log" class="Str"() -> ("Value"=w123:string)  [unwired: 2 in, 2 out]
                      n310 = Concatenate Strings(w123, w122) -> (w121:string)
                      n311 = property on="Serial log" class="Str"("Value"=w121) -> ()  [unwired: 2 in, 2 out]
                    }
                  }
                }
                frame Error {
                }
              }
              n312 = property on="stop" class="Bool (strict)"() -> ("Value"=w112:bool)  [unwired: 2 in, 2 out]
            }
          }
        }
        n313 = property on="Baud Rate" class="DigNum (strict)"("DisabledEnum"=w107) -> ()  [unwired: 2 in, 2 out]
      }
      frame "Clean up" {
        w632 = refnum<k16> refnum  # Empty UDP Socket
        n314 = property on="UDP Socket" class="Ref (strict)"() -> ("Value"=w630:refnum<k16>)  [unwired: 2 in, 2 out]
        n315 = Equal?(x=w630, y=w632) -> (x = y?=w631:bool)
        n316 = case shown="False" w631 {
          tunnel: w630 -> [_ w639]
          tunnel: [errorcluster {"status"=FALSE, "code"=0, "source"=""} ("error out") w638] -> w623
          frame False {
          }
          frame True {
            n317 = UDP Close(connection ID=w639) -> (error out=w638:errorcluster)  [unwired: 1 in, 1 out]
          }
        }
        n318 = property on="WiFi Network" class="Bool (strict)"() -> ("Value"=w626:bool)  [unwired: 2 in, 2 out]
        n319 = case shown="True" w626 {
          tunnel: [errorcluster {"status"=FALSE, "code"=0, "source"=""} ("error out") w636] -> w624
          frame False {
          }
          frame True {
            n320 = call "Stop WiFi Hotspot.vi"() -> ("error out"=w636:errorcluster)  [unwired: 9 in, 2 out]
          }
        }
        n321 = property on="UDP Socket" class="Bool (strict)"(error in=w623, "Value"=FALSE ("UDP Communication")) -> ()  [unwired: 1 in, 2 out]
        n322 = property on="Controller" class="TypRef (strict)"() -> ("Value"=w629:refnum<k1>)  [unwired: 2 in, 2 out]
        n323 = property on="WiFi Network" class="Bool (strict)"(error in=w624, "Value"=FALSE ("WiFi Network")) -> ()  [unwired: 1 in, 2 out]
        n324 = call-poly <vilib>:"Close Input Device.vi"("device ID"=w629) -> ("error out"=w621:errorcluster)  [unwired: 9 in]
        n325 = Merge Errors(w627, w621, w623, w624) -> (w628:errorcluster)
        n326 = property on="User controller" class="Bool (strict)"(error in=w621, "Value"=FALSE ("User controller")) -> ()  [unwired: 1 in, 2 out]
      }
      frame "Error" {
        n327 = while {
          tunnel: w640 -> [w646]
          tunnel: [w644] -> w641
          stop <- w645 stop-if-true
          n328 = flat-sequence {
            tunnel: w646 -> [w649]
            tunnel: [w649] -> w643
            tunnel: [w653] -> w645
            tunnel: [w650] -> w644
            tunnel: w643 -> [w657]
            frame #0 {
              n329 = property on="restart" class="Bool (strict)"("Visible"=TRUE, "DisabledEnum"=T5."Enabled" ("Disabled")) -> ()  [unwired: 2 in, 2 out]
            }
            frame #1 {
              w656 = T7 0 items=["no dialog", "OK message", "continue or stop message", "OK message + warnings", "continue/stop + warnings"] ("type of dialog (OK msg:1)")
              n330 = call <vilib>:"General Error Handler.vi"("[user-defined codes]"=i32[] [-8000], "[user-defined descriptions]"=string[] ["WiFi password must be of 8 to 63 characters"], "type of dialog (OK msg:1)"=w656, "error in (no error)"=w657) -> ()  [unwired: 7 in, 5 out]
              n331 = property on="stop" class="Bool (strict)"() -> ("Value"=w654:bool)  [unwired: 2 in, 2 out]
              n332 = Build Array("restart", w654) -> (w651:bool[])
              n333 = Or(x="restart", y=w654) -> (x .or. y?=w653:bool)
              n334 = Boolean Array To Number(Boolean array=w651) -> (number=w652:u32)
              n335 = case shown="1" w652 {
                tunnel: [enum16{"Start up", "Error", "Main", "Clean up"}."Clean up" enum16{"Start up", "Error", "Main", "Clean up"}."Start up"] -> w650
                frame 2, Default {
                }
                frame 1 {
                  n336 = property on="Controller" class="TypRef (strict)"() -> ("Value"=w661:refnum<k1>)  [unwired: 2 in, 2 out]
                  n337 = call-poly <vilib>:"Close Input Device.vi"("device ID"=w661) -> ()  [unwired: 9 in, 1 out]
                }
              }
            }
          }
        }
      }
    }
  }
  n338 = flat-sequence {
    tunnel: w3 -> [_]
    tunnel: w2 -> [w663]
    frame #0 {
      n339 = property class="App"() -> ("App.Kind"=w664:T8)  [unwired: 2 in, 2 out]
      n340 = case shown="\"Run Time System\"" w664 {
        frame Default {
        }
        frame "Run Time System" {
          n341 = Quit LabVIEW() -> ()  [unwired: 1 in]
        }
      }
      "Error Out" <- w663
    }
  }
